vi "pp3_DAQinit.vi"(8 "error in (no error)":errorcluster, 11 "Daq config in":T1={"Sound AO"="Dev6/ao0", "Shock intesity AO"="Dev6/ao1", "Code_LED DO"="Dev6/port1:2", "Switch DI"="Dev6/port0/line0", "Webcam"="cam9", "Sound AO task"="", "Sound card task"=0, "Shock intensity AO task"="", "Code_LED DO task"="", "Switch DI task"="", "AO <=> Sound card"=FALSE, "Sound card"=0, "sample rate"=100000.0, "Variable shock"=TRUE, "Webcam on"=FALSE, "Waveform memo"={"t0"=timestamp(0 s since 1904-01-01), "dt"=1.0, "Y"=[]}, "First time"=FALSE, "Tone trigger"="PFI1"} {"sample rate" min=8000.0; "Sound card task" format="%.0x"}) -> (0 "error out":errorcluster={"status"=FALSE, "code"=0, "source"="\n"}, 3 "Daq config out":T1={"Sound AO"="Dev6/ao0", "Shock intesity AO"="Dev6/ao1", "Code_LED DO"="Dev6/port1:2", "Switch DI"="Dev6/port0/line0", "Webcam"="cam9", "Sound AO task"="", "Sound card task"=0, "Shock intensity AO task"="", "Code_LED DO task"="", "Switch DI task"="", "AO <=> Sound card"=FALSE, "Sound card"=0, "sample rate"=100000.0, "Variable shock"=TRUE, "Webcam on"=FALSE, "Waveform memo"={"t0"=timestamp(0 s since 1904-01-01), "dt"=1.0, "Y"=[]}, "First time"=FALSE, "Tone trigger"="PFI1"} {"sample rate" min=8000.0; "Sound card task" format="%.0x"})   [LabVIEW 2013]
uses:
  pp3_CTL_DaqConfig.ctl
  <vilib>/userdefined/High Color/IMAQdx.ctl
  <vilib>/sound2/lvsound2.llb/Sound Output Task ID.ctl
  <vilib>/sound2/lvsound2.llb/Sampling Mode.ctl
  <vilib>/sound2/lvsound2.llb/Sound Data Format.ctl
  <vilib>/DAQmx/create/channels.llb/DAQmx Create Channel (DO-Digital Output).vi
  <vilib>/DAQmx/create/channels.llb/DAQmx Create Channel (DI-Digital Input).vi
  <vilib>/DAQmx/create/channels.llb/DAQmx Create Channel (AO-Voltage-Basic).vi
  <vilib>/DAQmx/configure/timing.llb/DAQmx Timing (Sample Clock).vi
  <resource>/objmgr/daqmx.rc
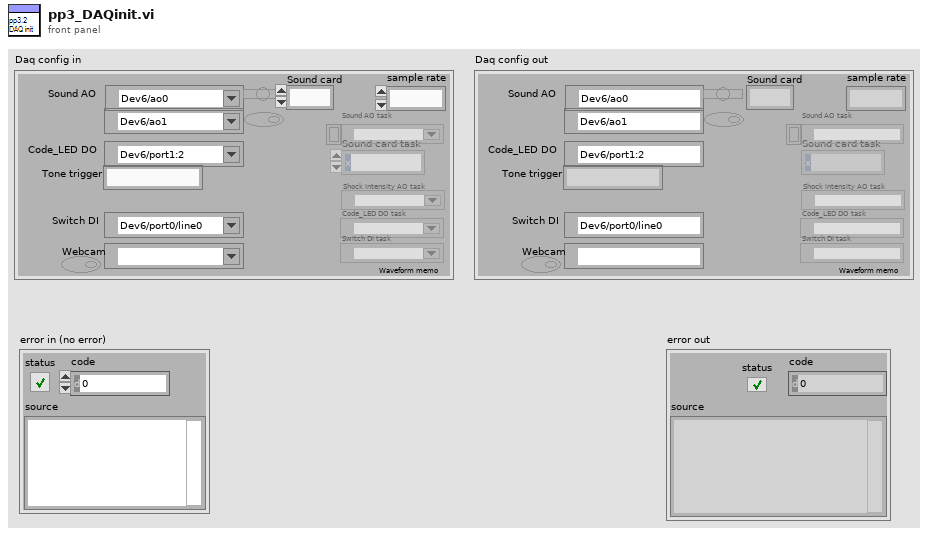
[diagram p1: front panel]
types:
  T1 = typedef "pp3_CTL_DaqConfig.ctl" = cluster{"Sound AO":tag, "Shock intesity AO":tag, "Code_LED DO":tag, "Switch DI":tag, "Webcam":T2, "Sound AO task":refnum<k21>, "Sound card task":T3, "Shock intensity AO task":refnum<k21>, "Code_LED DO task":refnum<k21>, "Switch DI task":refnum<k21>, "AO <=> Sound card":bool, "Sound card":u32, "sample rate":dbl, "Variable shock":bool, "Webcam on":bool, "Waveform memo":waveform(dbl), "First time":bool, "Tone trigger":string}
  T2 = typedef "IMAQdx.ctl" = refnum<k21>
  T3 = typedef "Sound Output Task ID.ctl" = u32
  T4 = typedef "Sound Data Format.ctl" = cluster{"sample rate (S/s)":dbl, "number of channels":i32, "bits per sample":i32}
  T5 = typedef "Sampling Mode.ctl" = i32
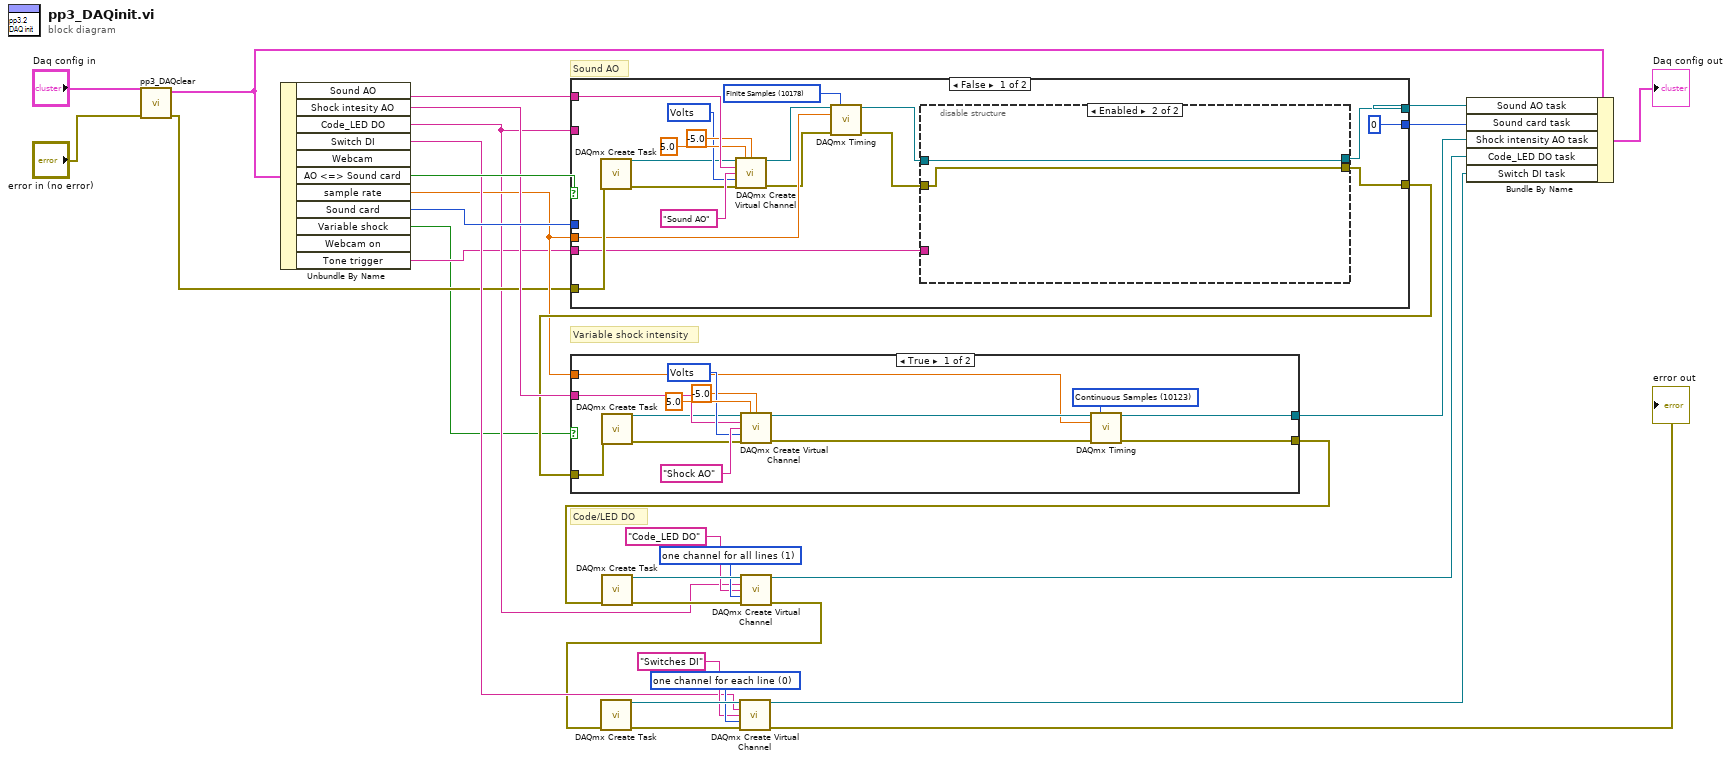
[diagram p0: block diagram]
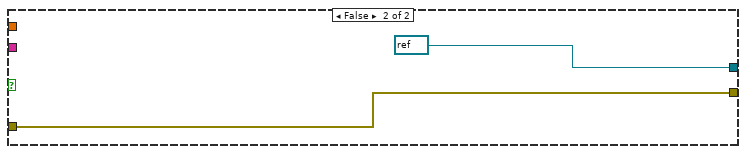
[diagram p2: hidden frame]
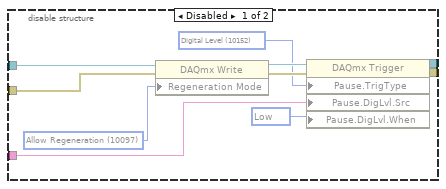
[diagram p3: hidden frame]
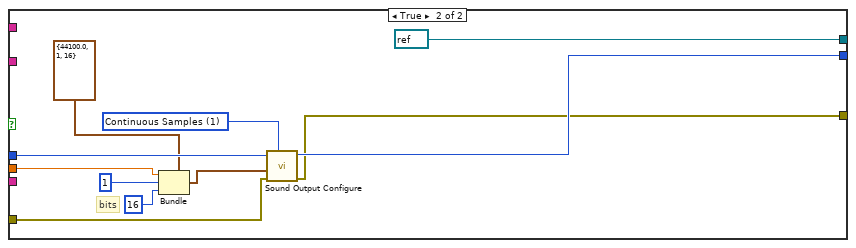
[diagram p4: hidden frame]
diagram:
  w17 = 0 items=["one channel for each line", "one channel for all lines"] ("line grouping")
  w21 = 1 items=["one channel for each line", "one channel for all lines"] ("line grouping")
  # "Code/LED DO"
  # "Variable shock intensity"
  # "Sound AO"
  n1 = call "pp3_DAQclear.vi"("error in (no error)"="error in (no error)", "Daq config in"="Daq config in") -> ("error out"=w4:errorcluster, "Daq config out"=w6:T1)  [unwired: 8 in]
  n2 = Unbundle By Name(w6) -> ("Sound AO"=w30:tag, "Shock intesity AO"=w25:tag, "Code_LED DO"=w3:tag, "Switch DI"=w15:tag, "AO <=> Sound card"=w31:bool, "sample rate"=w8:dbl, "Sound card"=w27:u32, "Variable shock"=w1:bool, "Tone trigger"=w2:string)  [unwired: 2 out]
  n3 = case shown="False" w31 {
    tunnel: w30 -> [w49 _]
    tunnel: [w39 refnum<k21> refnum ("task out")] -> w28
    tunnel: w27 -> [_ w71]
    tunnel: [T3 0 ("task ID") w67] -> w26
    tunnel: w4 -> [w43 w66]
    tunnel: [w38 w65] -> w12
    tunnel: w8 -> [w36 w64]
    tunnel: w3 -> [_ _]
    tunnel: w2 -> [w40 _]
    frame False {
      w33 = 10178 items=["Finite Samples"=10178, "Continuous Samples"=10123, "Hardware Timed Single Point"=12522] ("sample mode")
      w44 = 10348 items=["Volts"=10348, "From Custom Scale"=10065] ("units")
      n4 = call <vilib>:"DAQmx Create Task.vi"("error in"=w43) -> ("task out"=w42:refnum<k21>, "error out"=w41:errorcluster)  [unwired: 13 in]
      n5 = call-poly <vilib>:"DAQmx Create Virtual Channel.vi"("task in"=w42, "maximum value"=5.0, "minimum value"=-5.0, "physical channels"=w49, "name to assign"="Sound AO", "units"=w44, "error in"=w41) -> ("task out"=w37:refnum<k21>, "error out"=w35:errorcluster)  [unwired: 7 in]
      n6 = call-poly <vilib>:"DAQmx Timing.vi"("task/channels in"=w37, "sample mode"=w33, "rate"=w36, "error in"=w35) -> ("task out"=w32:refnum<k21>, "error out"=w34:errorcluster)  [unwired: 10 in]
      n7 = disable-structure shown="Enabled" {
        disable-tunnel: w32 -> [w58 w61]
        disable-tunnel: w34 -> [w57 w60]
        disable-tunnel: w40 -> [w53 _]
        disable-tunnel: [w51 w61] -> w39
        disable-tunnel: [w50 w60] -> w38
        frame Disabled {
          w56 = 10214 items=["High"=10192, "Low"=10214] ("Pause.DigLvl.When")
          w52 = 10152 items=["Analog Level"=10101, "Analog Window"=10103, "Digital Level"=10152, "Digital Pattern"=10398, "None"=10230] ("Pause.TrigType")
          w59 = 10097 items=["Allow Regeneration"=10097, "Do Not Allow Regeneration"=10158] ("RegenMode")
          n8 = property class="DAQmx Write"(reference=w58, error in=w57, "Regeneration Mode"=w59) -> (reference out=w55:refnum<k21>, error out=w54:errorcluster)
          n9 = property class="DAQmx Trigger"(reference=w55, error in=w54, "Pause.TrigType"=w52, "Pause.DigLvl.Src"=w53, "Pause.DigLvl.When"=w56) -> (reference out=w51:refnum<k21>, error out=w50:errorcluster)
        }
        frame Enabled {
        }
      }
    }
    frame True {
      w70 = T5 1 items=["Finite Samples", "Continuous Samples"] ("sample mode")
      # "bits"
      n10 = Bundle(cluster=T4 {"sample rate (S/s)"=44100.0, "number of channels"=1, "bits per sample"=16} ("sound format"), "sample rate (S/s)"=w64, "number of channels"=1 ("Input.BufSize"), "bits per sample"=16 ("Input.BufSize")) -> (w62:T4)
      n11 = call <vilib>:"Sound Output Configure.vi"("sample mode"=w70, "error in (no error)"=w66, "sound format"=w62, "device ID"=w71) -> ("error out"=w65:errorcluster, "task ID"=w67:T3)  [unwired: 6 in]
    }
  }
  n12 = case shown="True" w1 {
    tunnel: w25 -> [w83 _]
    tunnel: [w77 refnum<k21> refnum ("task out")] -> w24
    tunnel: w8 -> [w79 _]
    tunnel: w12 -> [w75 w88]
    tunnel: [w76 w88] -> w11
    frame True {
      w78 = 10123 items=["Finite Samples"=10178, "Continuous Samples"=10123, "Hardware Timed Single Point"=12522] ("sample mode")
      w84 = 10348 items=["Volts"=10348, "From Custom Scale"=10065] ("units")
      n13 = call <vilib>:"DAQmx Create Task.vi"("error in"=w75) -> ("task out"=w73:refnum<k21>, "error out"=w74:errorcluster)  [unwired: 13 in]
      n14 = call-poly <vilib>:"DAQmx Create Virtual Channel.vi"("task in"=w73, "maximum value"=5.0, "minimum value"=-5.0, "physical channels"=w83, "name to assign"="Shock AO", "units"=w84, "error in"=w74) -> ("task out"=w81:refnum<k21>, "error out"=w80:errorcluster)  [unwired: 7 in]
      n15 = call-poly <vilib>:"DAQmx Timing.vi"("task/channels in"=w81, "sample mode"=w78, "rate"=w79, "error in"=w80) -> ("task out"=w77:refnum<k21>, "error out"=w76:errorcluster)  [unwired: 10 in]
    }
    frame False {
    }
  }
  n16 = call <vilib>:"DAQmx Create Task.vi"("error in"=w11) -> ("task out"=w22:refnum<k21>, "error out"=w23:errorcluster)  [unwired: 13 in]
  n17 = call-poly <vilib>:"DAQmx Create Virtual Channel.vi"("task in"=w22, "lines"=w3, "name to assign"="Code_LED DO", "line grouping"=w21, "error in"=w23) -> ("task out"=w14:refnum<k21>, "error out"=w10:errorcluster)  [unwired: 9 in]
  n18 = call <vilib>:"DAQmx Create Task.vi"("error in"=w10) -> ("task out"=w18:refnum<k21>, "error out"=w19:errorcluster)  [unwired: 13 in]
  n19 = call-poly <vilib>:"DAQmx Create Virtual Channel.vi"("task in"=w18, "lines"=w15, "name to assign"="Switches DI", "line grouping"=w17, "error in"=w19) -> ("task out"=w13:refnum<k21>, "error out"=→"error out":errorcluster)  [unwired: 9 in]
  n20 = Bundle By Name(cluster=w6, "Sound AO task"=w28, "Sound card task"=w26, "Shock intensity AO task"=w24, "Code_LED DO task"=w14, "Switch DI task"=w13) -> (→"Daq config out":T1)
